vi "Heater_Enable_Chs.vi"() -> (0 "Bus Bar 4":T1={"Bus Bar"="EnFlo_Tunnel:Bus Bar 1 Enable:Y-ve Top", "Connected Items"=[]}, 1 "Bus Bar 3":T1={"Bus Bar"="EnFlo_Tunnel:Bus Bar 1 Enable:Y-ve Top", "Connected Items"=[]}, 2 "Bus Bar 2":T1={"Bus Bar"="EnFlo_Tunnel:Bus Bar 1 Enable:Y-ve Top", "Connected Items"=[]}, 3 "Bus Bar 1":T1={"Bus Bar"="EnFlo_Tunnel:Bus Bar 1 Enable:Y-ve Top", "Connected Items"=[]}, 4 "Wanted if these channels are great than zero":string[](array[string])=["EnFlo_Tunnel:Power:Chiller_Pump_Floor", "EnFlo_Tunnel:Power:Chiller_Pump_Exchanger", "EnFlo_Tunnel:Power:Exit_Heaters", "EnFlo_Tunnel:Enable:Inlet_Lamps"], 5 "Inlet Heaters":T1={"Bus Bar"="", "Connected Items"=["EnFlo_Tunnel:Enable:Inlet_Y=0_Z=50", "EnFlo_Tunnel:Enable:Inlet_Y=0_Z=150", "EnFlo_Tunnel:Enable:Inlet_Y=0_Z=250", "EnFlo_Tunnel:Enable:Inlet_Y=0_Z=350", "EnFlo_Tunnel:Enable:Inlet_Y=0_Z=450", "EnFlo_Tunnel:Enable:Inlet_Y=0_Z=550", "EnFlo_Tunnel:Enable:Inlet_Y=0_Z=650", "EnFlo_Tunnel:Enable:Inlet_Y=0_Z=750", "EnFlo_Tunnel:Enable:Inlet_Y=0_Z=850", "EnFlo_Tunnel:Enable:Inlet_Y=0_Z=950", "EnFlo_Tunnel:Enable:Inlet_Y=0_Z=1050", "EnFlo_Tunnel:Enable:Inlet_Y=0_Z=1150", "EnFlo_Tunnel:Enable:Inlet_Y=0_Z=1250", "EnFlo_Tunnel:Enable:Inlet_Y=0_Z=1350", "EnFlo_Tunnel:Enable:Inlet_Y=0_Z=1450"]})   [LabVIEW 2017]
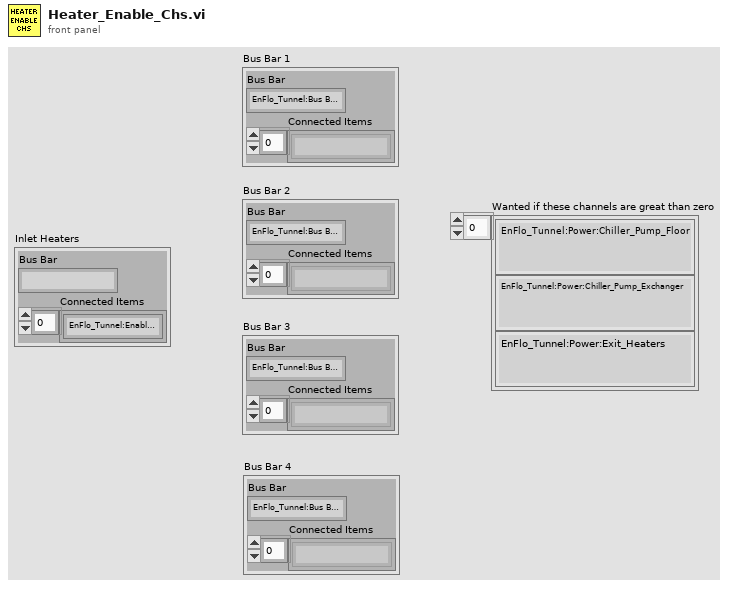
[diagram p1: front panel]
types:
  T1 = cluster{"Bus Bar":string, "Connected Items":string[]}
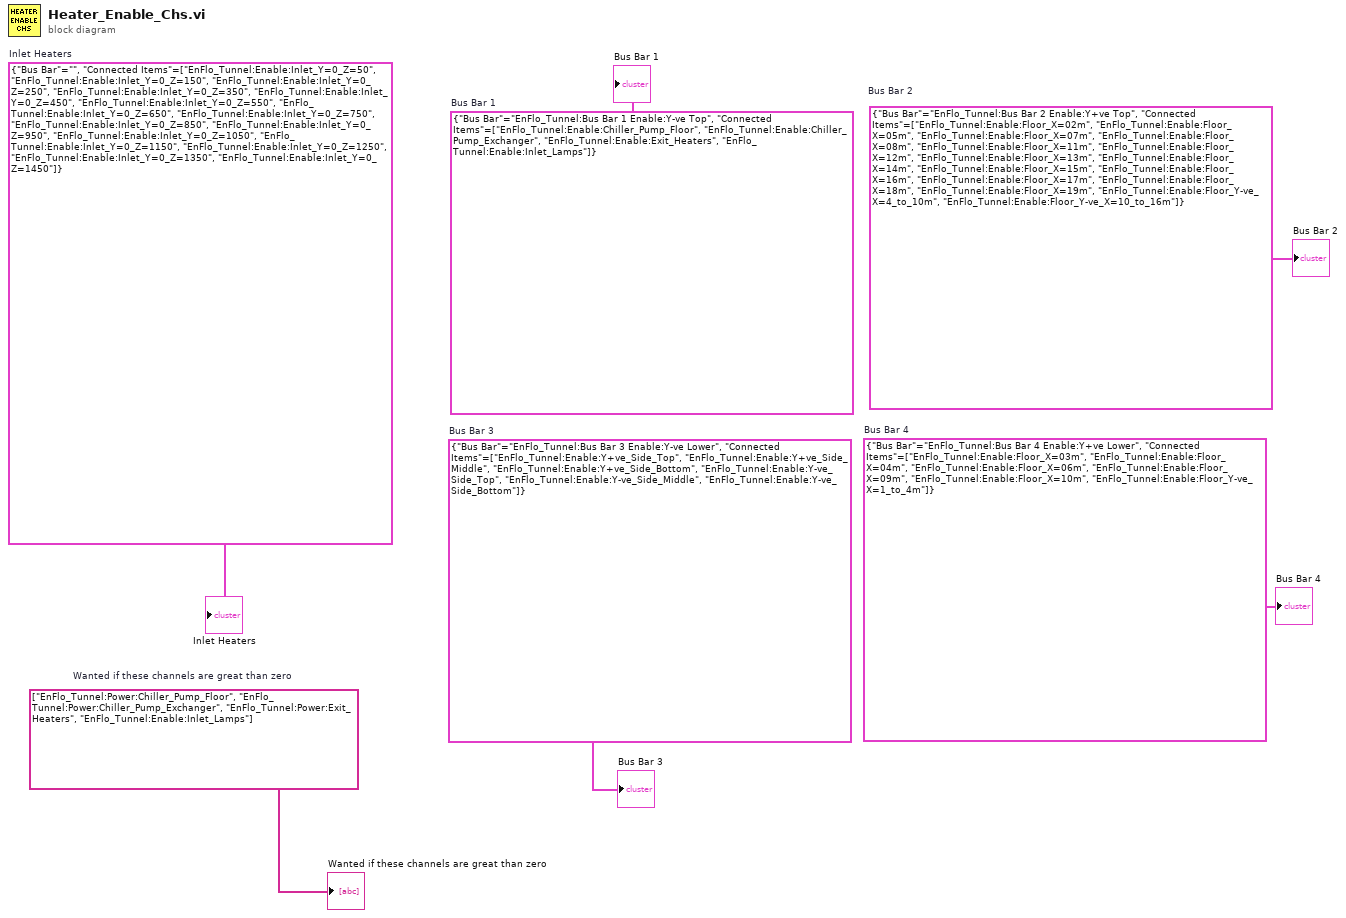
[diagram p0: block diagram]
diagram:
  w1 = string[] ["EnFlo_Tunnel:Power:Chiller_Pump_Floor", "EnFlo_Tunnel:Power:Chiller_Pump_Exchanger", "EnFlo_Tunnel:Power:Exit_Heaters", "EnFlo_Tunnel:Enable:Inlet_Lamps"]  # Wanted if these channels are great than zero
  w2 = T1 {"Bus Bar"="", "Connected Items"=["EnFlo_Tunnel:Enable:Inlet_Y=0_Z=50", "EnFlo_Tunnel:Enable:Inlet_Y=0_Z=150", "EnFlo_Tunnel:Enable:Inlet_Y=0_Z=250", "EnFlo_Tunnel:Enable:Inlet_Y=0_Z=350", "EnFlo_Tunnel:Enable:Inlet_Y=0_Z=450", "EnFlo_Tunnel:Enable:Inlet_Y=0_Z=550", "EnFlo_Tunnel:Enable:Inlet_Y=0_Z=650", "EnFlo_Tunnel:Enable:Inlet_Y=0_Z=750", "EnFlo_Tunnel:Enable:Inlet_Y=0_Z=850", "EnFlo_Tunnel:Enable:Inlet_Y=0_Z=950", "EnFlo_Tunnel:Enable:Inlet_Y=0_Z=1050", "EnFlo_Tunnel:Enable:Inlet_Y=0_Z=1150", "EnFlo_Tunnel:Enable:Inlet_Y=0_Z=1250", "EnFlo_Tunnel:Enable:Inlet_Y=0_Z=1350", "EnFlo_Tunnel:Enable:Inlet_Y=0_Z=1450"]}  # Inlet Heaters
  w3 = T1 {"Bus Bar"="EnFlo_Tunnel:Bus Bar 3 Enable:Y-ve Lower", "Connected Items"=["EnFlo_Tunnel:Enable:Y+ve_Side_Top", "EnFlo_Tunnel:Enable:Y+ve_Side_Middle", "EnFlo_Tunnel:Enable:Y+ve_Side_Bottom", "EnFlo_Tunnel:Enable:Y-ve_Side_Top", "EnFlo_Tunnel:Enable:Y-ve_Side_Middle", "EnFlo_Tunnel:Enable:Y-ve_Side_Bottom"]}  # Bus Bar 3
  w4 = T1 {"Bus Bar"="EnFlo_Tunnel:Bus Bar 4 Enable:Y+ve Lower", "Connected Items"=["EnFlo_Tunnel:Enable:Floor_X=03m", "EnFlo_Tunnel:Enable:Floor_X=04m", "EnFlo_Tunnel:Enable:Floor_X=06m", "EnFlo_Tunnel:Enable:Floor_X=09m", "EnFlo_Tunnel:Enable:Floor_X=10m", "EnFlo_Tunnel:Enable:Floor_Y-ve_X=1_to_4m"]}  # Bus Bar 4
  w5 = T1 {"Bus Bar"="EnFlo_Tunnel:Bus Bar 2 Enable:Y+ve Top", "Connected Items"=["EnFlo_Tunnel:Enable:Floor_X=02m", "EnFlo_Tunnel:Enable:Floor_X=05m", "EnFlo_Tunnel:Enable:Floor_X=07m", "EnFlo_Tunnel:Enable:Floor_X=08m", "EnFlo_Tunnel:Enable:Floor_X=11m", "EnFlo_Tunnel:Enable:Floor_X=12m", "EnFlo_Tunnel:Enable:Floor_X=13m", "EnFlo_Tunnel:Enable:Floor_X=14m", "EnFlo_Tunnel:Enable:Floor_X=15m", "EnFlo_Tunnel:Enable:Floor_X=16m", "EnFlo_Tunnel:Enable:Floor_X=17m", "EnFlo_Tunnel:Enable:Floor_X=18m", "EnFlo_Tunnel:Enable:Floor_X=19m", "EnFlo_Tunnel:Enable:Floor_Y-ve_X=4_to_10m", "EnFlo_Tunnel:Enable:Floor_Y-ve_X=10_to_16m"]}  # Bus Bar 2
  w6 = T1 {"Bus Bar"="EnFlo_Tunnel:Bus Bar 1 Enable:Y-ve Top", "Connected Items"=["EnFlo_Tunnel:Enable:Chiller_Pump_Floor", "EnFlo_Tunnel:Enable:Chiller_Pump_Exchanger", "EnFlo_Tunnel:Enable:Exit_Heaters", "EnFlo_Tunnel:Enable:Inlet_Lamps"]}  # Bus Bar 1
  "Bus Bar 1" <- w6
  "Bus Bar 2" <- w5
  "Bus Bar 4" <- w4
  "Bus Bar 3" <- w3
  "Inlet Heaters" <- w2
  "Wanted if these channels are great than zero" <- w1
